vi "writeI8.vi"(8 "error in (no error)":errorcluster, 10 "Input":i8, 11 "ModbusBuffer in":refnum<class "ModbusBuffer.lvclass">) -> (0 "error out":errorcluster, 3 "ModbusBuffer out":refnum<class "ModbusBuffer.lvclass">)   [LabVIEW 2016, in "RTModbus.lvlib" / "ModbusBuffer.lvclass"]
uses:
  ModbusBuffer.lvclass
  ModbusBuffer.lvclass/ModbusBuffer.ctl
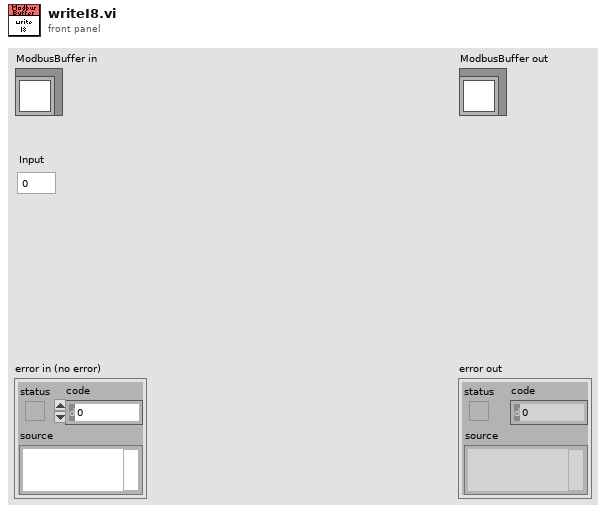
[diagram p1: front panel]
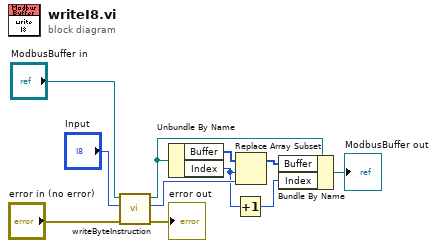
[diagram p0: block diagram]
diagram:
  n1 = call "writeByteInstruction.vi"("error in (no error)"="error in (no error)", "Input"="Input", "ModbusBuffer in"="ModbusBuffer in") -> ("error out"=→"error out":errorcluster, "Output"=w8:u16, "ModbusBuffer out"=w4:refnum<class "ModbusBuffer.lvclass">)  [unwired: 6 in]
  n2 = Unbundle By Name(w4) -> ("Buffer"=w5:u16[], "Index"=w2:i32)
  n3 = Increment(x=w2) -> (x+1=w1:i32)
  n4 = Replace Array Subset(array=w5, new element=w8, index=w2) -> (w11:u16[])
  n5 = Bundle By Name(cluster=w4, "Buffer"=w11, "Index"=w1) -> (→"ModbusBuffer out":refnum<class "ModbusBuffer.lvclass">)
